vi "Clean Build Artifacts.vi"(0 "NI Build Specification in":refnum<class "Executable_LV.lvclass">, 11 "error in (no error)":errorcluster) -> (4 "NI Build Specification out":refnum<class "Executable_LV.lvclass">, 15 "error out":errorcluster)   [LabVIEW 2017, in "CL_G3_VIComponentBuilder.lvlib" / "Executable_LV.lvclass"]
doc: "Deletes the executable at the location specified by the Output Directory in the build spec."
uses:
  Executable_LV.lvclass
  C:/Tool Chain Support/Software Module Builder/Source/Exports/NI Build Specification_LV/NI Build Specification_LV.lvclass
  <vilib>/AppBuilder/AB_API/common/AB_API Build Object Selector.ctl
  NI Build Specification_LV/NI Build Specification_LV.lvclass/NI Build Specification_LV.ctl
  NI Build Specification_LV/Accessors/Read TargetRef Containting Build Spec.vi
  NI Build Specification_LV/Accessors/Read Project Reference.vi
  NI Build Specification_LV/Accessors/Read Export's Build Spec Name.vi
  <vilib>/AppBuilder/AB_API/Build/NI_AB_API_Build.lvclass
  NI Build Specification_LV/NI Build Specification_LV.lvclass
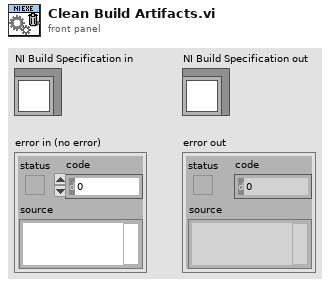
[diagram p1: front panel]
types:
  T1 = typedef "AB_API Build Object Selector.ctl" = enum16{"Source Distribution", "Deployable Source Distribution", "DLL", "EXE", "Packed Library", "Deployable Packed Library", "RT EXE", ".NET Interop Assembly"}
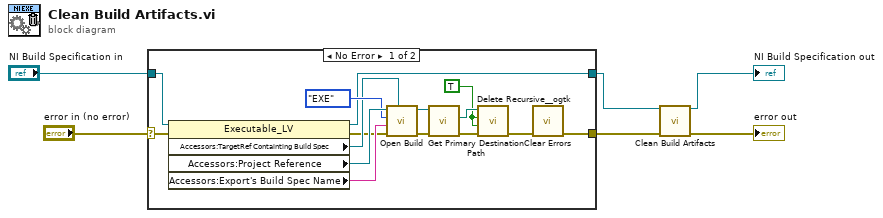
[diagram p0: block diagram]
diagram:
  n1 = case shown="No Error" "error in (no error)" {
    selector: "error in (no error)" -> [w14 w22]
    tunnel: "NI Build Specification in" -> [w19 w23]
    tunnel: [w18 w23] -> w2
    tunnel: [w7 w22] -> w4
    frame No Error {
      w10 = TRUE ("Ignore Read-Only? (FALSE)")
      n2 = property class="Executable_LV"(reference=w19, error in=w14) -> (reference out=w18:refnum<class "Executable_LV.lvclass">, error out=w13:errorcluster, "Accessors:TargetRef Containting Build Spec"=w16:refnum<vi>, "Accessors:Project Reference"=w21:refnum<vi>, "Accessors:Export's Build Spec Name"=w15:string)
      n3 = call <vilib>:"Open Build.vi"("TargetItem Refnum"=w16, "error in (no error)"=w13, "Build specification name"=w15, "Build object selector"=AB_API_Build_Object_Selector."EXE", "Project Refnum"=w21) -> ("error out"=w12:errorcluster, "NI_AB_API_Build out"=w17:refnum<class "NI_AB_API_Build.lvclass">)  [unwired: 5 in]
      n4 = call-dynamic "Get Primary Destination Path.vi"("error in (no error)"=w12, "NI_AB_API_Build in"=w17) -> ("error out"=w9:errorcluster, "Primary destination path"=w11:path)  [unwired: 7 in, 1 out]
      n5 = call <userlib>:"Delete Recursive__ogtk.vi"("error in (no error)"=w9, "Ignore Read-Only? (FALSE)"=w10, "Recursive? (FALSE)"=w10, "Path"=w11) -> ("error out"=w8:errorcluster)  [unwired: 6 in, 1 out]
      n6 = call <vilib>:"Clear Errors.vi"("error in (no error)"=w8) -> ("error out"=w7:errorcluster)  [unwired: 5 in, 1 out]
    }
    frame Error {
    }
  }
  n7 = call-parent "Clean Build Artifacts.vi"("NI Build Specification in"=w2, "error in (no error)"=w4) -> ("NI Build Specification out"=→"NI Build Specification out":refnum<class "Executable_LV.lvclass">, "error out"=→"error out":errorcluster)  [unwired: 12 in]
